vi "S706 disable voltage.vi"(8 "error in (no error)":errorcluster) -> (0 "error out":errorcluster)   [LabVIEW 2014]
uses:
  <vilib>/CANopenLib/CANOPEN.llb/CANopen SDO Create.vi
  <vilib>/CANopenLib/CANOPEN.llb/CANopen SDO Write [U16].vi
  <vilib>/CANopenLib/CANOPEN.llb/CANopen SDO Close.vi
  <vilib>/CANopenLib/CANOPEN.llb/CANopen Interface Close.vi
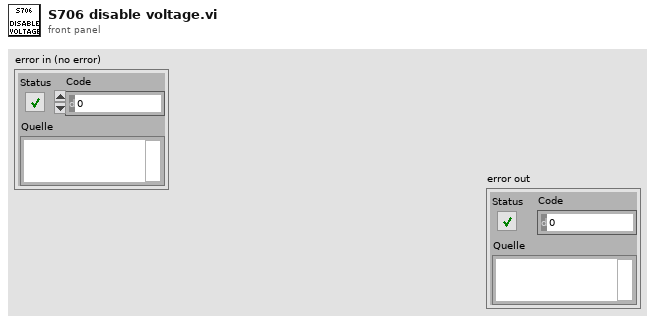
[diagram p1: front panel]
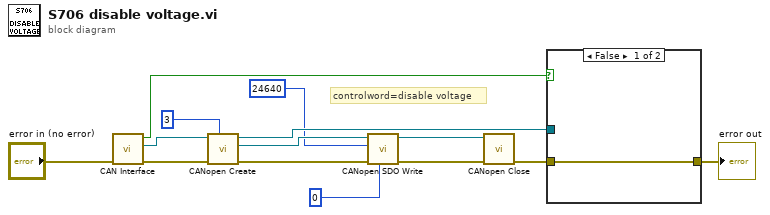
[diagram p0: block diagram]
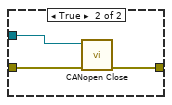
[diagram p2: hidden frame]
diagram:
  # "controlword=disable voltage"
  n1 = call "CAN Interface.vi"("error in (no error)"="error in (no error)") -> ("error out"=w2:errorcluster, "interface object out"=w3:refnum<k20>, "Interface schließen?"=w4:bool)  [unwired: 8 in]
  n2 = call-poly <vilib>:"CANopen Create.vi"("node-ID"=u8 3, "error in (no error)"=w2, "interface object in"=w3) -> ("error out"=w5:errorcluster, "SDO object out"=w11:refnum<k20>, "interface object out"=w10:refnum<k20>)  [unwired: 6 in]
  n3 = call-poly <vilib>:"CANopen SDO Write.vi"("U16 data"=u16 0, "error in (no error)"=w5, "object index"=u16 24640, "SDO object in"=w11) -> ("error out"=w13:errorcluster, "SDO object out"=w12:refnum<k20>)  [unwired: 5 in, 1 out]
  n4 = call-poly <vilib>:"CANopen Close.vi"("error in (no error)"=w13, "SDO object in"=w12) -> ("error out"=w9:errorcluster)  [unwired: 9 in]
  n5 = case shown="False" w4 {
    tunnel: w10 -> [_ w18]
    tunnel: w9 -> [w15 w17]
    tunnel: [w15 w16] -> w8
    frame False {
    }
    frame True {
      n6 = call-poly <vilib>:"CANopen Close.vi"("error in (no error)"=w17, "interface object in"=w18) -> ("error out"=w16:errorcluster)  [unwired: 9 in]
    }
  }
  "error out" <- w8
